vi "Log Response Times.vi"() -> ()   [LabVIEW 2015]
uses:
  <vilib>/addons/zeromq/socket_type.ctl
  <userlib>/_OpenG.lib/array/array.llb/Delete Elements from 1D Array (DBL)__ogtk.vi
  <vilib>/Utility/file.llb/Write Delimited Spreadsheet (string).vi
  <vilib>/addons/zeromq/zmq_context.lvclass
  <vilib>/addons/zeromq/zeromq.lvlib
  <vilib>/addons/zeromq/zmq_socket.lvclass
panel:
  out "Event Read Times":cluster{dbl[], i32[]}(graph)={[0.0009271277813240886, 0.2630802224110812, 0.5252333170408383, 0.7873864116705954, 1.0495395063003525, 1.3116926009301095, 1.5738456955598668, 1.835998790189624, 2.098151884819381, 2.360304979449138, 2.622458074078895, 2.8846111687086524, 3.1467642633384094, 3.4089173579681664, 3.671070452597924, 3.933223547227681, 4.195376641857438, 4.457529736487195, 4.719682831116952, 4.981835925746709, 5.243989020376466, 5.506142115006224, 5.768295209635981, 6.030448304265738, 6.292601398895495, 6.554754493525252, 6.816907588155009, 7.079060682784766, 7.341213777414524, 7.603366872044281, 7.865519966674038, 8.127673061303794, 8.389826155933552, 8.65197925056331, 8.914132345193066, 9.176285439822824, 9.43843853445258, 9.700591629082338, 9.962744723712094, 10.224897818341852, 10.487050912971608, 10.749204007601366, 11.011357102231123, 11.27351019686088, 11.535663291490637, 11.797816386120394, 12.059969480750151, 12.322122575379908, 12.584275670009665, 12.846428764639423, 13.10858185926918, 13.370734953898937, 13.632888048528693, 13.895041143158451, 14.157194237788207, 14.419347332417965, 14.681500427047723, 14.94365352167748, 15.205806616307237, 15.467959710936993, 15.730112805566751, 15.992265900196507, 16.254418994826263, 16.516572089456023, 16.77872518408578, 17.040878278715535, 17.303031373345295, 17.56518446797505, 17.827337562604807, 18.089490657234563, 18.351643751864323, 18.61379684649408, 18.875949941123835, 19.138103035753595, 19.40025613038335, 19.662409225013107, 19.924562319642863, 20.186715414272623, 20.44886850890238, 20.711021603532135, 20.97317469816189, 21.23532779279165, 21.497480887421407, 21.759633982051163, 22.021787076680923, 22.28394017131068, 22.546093265940435, 22.80824636057019, 23.07039945519995, 23.332552549829707, 23.594705644459463, 23.856858739089223, 24.11901183371898, 24.381164928348735, 24.64331802297849, 24.90547111760825, 25.167624212238007, 25.429777306867763, 25.691930401497522, 25.95408349612728], [281, 0, 0, 2, 0, 0, 0, 0, 0, 0, 1, 1, 1, 4, 11, 42, 21, 22, 12, 28, 8, 21, 11, 13, 18, 15, 90, 33, 52, 42, 68, 35, 22, 24, 110, 9, 3, 4, 4, 0, 1, 7, 1, 2, 0, 1, 0, 0, 0, 2, 0, 0, 0, 0, 0, 0, 0, 0, 0, 1, 0, 0, 0, 2, 0, 0, 1, 0, 2, 3, 0, 1, 3, 0, 1, 0, 0, 0, 0, 0, 0, 0, 0, 0, 0, 0, 0, 0, 1, 0, 0, 0, 0, 0, 0, 1, 0, 0, 0, 0]}
  out "Error Read Times":cluster{dbl[], i32[]}(graph)={[0.0009430865757167339, 0.30094855814939364, 0.6009540297230705, 0.9009595012967475, 1.2009649728704244, 1.5009704444441012, 1.8009759160177783, 2.100981387591455, 2.400986859165132, 2.700992330738809, 3.0009978023124857, 3.3010032738861628, 3.60100874545984, 3.9010142170335165, 4.201019688607193, 4.501025160180871, 4.801030631754547, 5.101036103328224, 5.401041574901901, 5.701047046475578, 6.001052518049255, 6.301057989622932, 6.601063461196609, 6.901068932770285, 7.201074404343963, 7.50107987591764, 7.801085347491316, 8.101090819064993, 8.40109629063867, 8.701101762212348, 9.001107233786025, 9.301112705359701, 9.601118176933378, 9.901123648507054, 10.201129120080731, 10.501134591654408, 10.801140063228086, 11.101145534801763, 11.40115100637544, 11.701156477949116, 12.001161949522793, 12.30116742109647, 12.601172892670148, 12.901178364243824, 13.2011838358175, 13.501189307391178, 13.801194778964854, 14.10120025053853, 14.40120572211221, 14.701211193685886, 15.001216665259562, 15.301222136833239, 15.601227608406916, 15.901233079980592, 16.20123855155427, 16.501244023127946, 16.801249494701622, 17.1012549662753, 17.40126043784898, 17.701265909422656, 18.001271380996332, 18.30127685257001, 18.601282324143686, 18.901287795717362, 19.20129326729104, 19.501298738864715, 19.801304210438392, 20.10130968201207, 20.401315153585745, 20.701320625159422, 21.0013260967331, 21.30133156830678, 21.601337039880455, 21.901342511454132, 22.20134798302781, 22.501353454601485, 22.801358926175162, 23.10136439774884, 23.401369869322515, 23.701375340896192, 24.00138081246987, 24.301386284043545, 24.60139175561722, 24.9013972271909, 25.20140269876458, 25.501408170338255, 25.80141364191193, 26.10141911348561, 26.401424585059285, 26.70143005663296, 27.00143552820664, 27.301440999780315, 27.60144647135399, 27.901451942927668, 28.201457414501345, 28.50146288607502, 28.8014683576487, 29.10147382922238, 29.401479300796055, 29.70148477236973], [281, 3, 0, 1, 0, 0, 0, 0, 0, 0, 3, 6, 4, 47, 33, 22, 47, 11, 11, 21, 8, 12, 25, 101, 51, 61, 65, 38, 35, 107, 13, 8, 3, 0, 1, 0, 4, 2, 0, 0, 0, 0, 0, 1, 0, 0, 1, 0, 0, 0, 0, 0, 1, 0, 0, 0, 1, 1, 1, 1, 0, 0, 0, 1, 0, 1, 0, 1, 0, 0, 0, 0, 0, 0, 0, 0, 0, 0, 0, 0, 0, 1, 0, 1, 0, 0, 0, 0, 0, 2, 0, 0, 0, 0, 0, 0, 0, 0, 0, 0]}
  in  "READ":bool
  in  "Error Log Request":string="{\"msg_id\":\"666\",\"msg_type\":\"get\",\"msg_property\":\"error\",\"XXX\":\"XXX\"}"
  in  "Event Log Request":string="{\"msg_id\":\"555\",\"msg_type\":\"get\",\"msg_property\":\"event\",\"XXX\":\"XXX\"}"
  in  "Message":string="{\"msg_id\":\"555\",\"msg_type\":\"read\",\"msg_property\":\"vmon\",\"8-04\":\"XXX\"}"
  in  "timeout (ms)":i32=1000
  in  "file":path=path "C:/Users/ANNIE/Documents/Logs/ZMQ_Read_Times.csv"
  in  "SEND":bool
  out "HB":bool
  out "error out":errorcluster
  in  "stop":bool
  in  "ZMQ endpoint":string="tcp://127.0.0.1:5555"
  out "REPLY":string
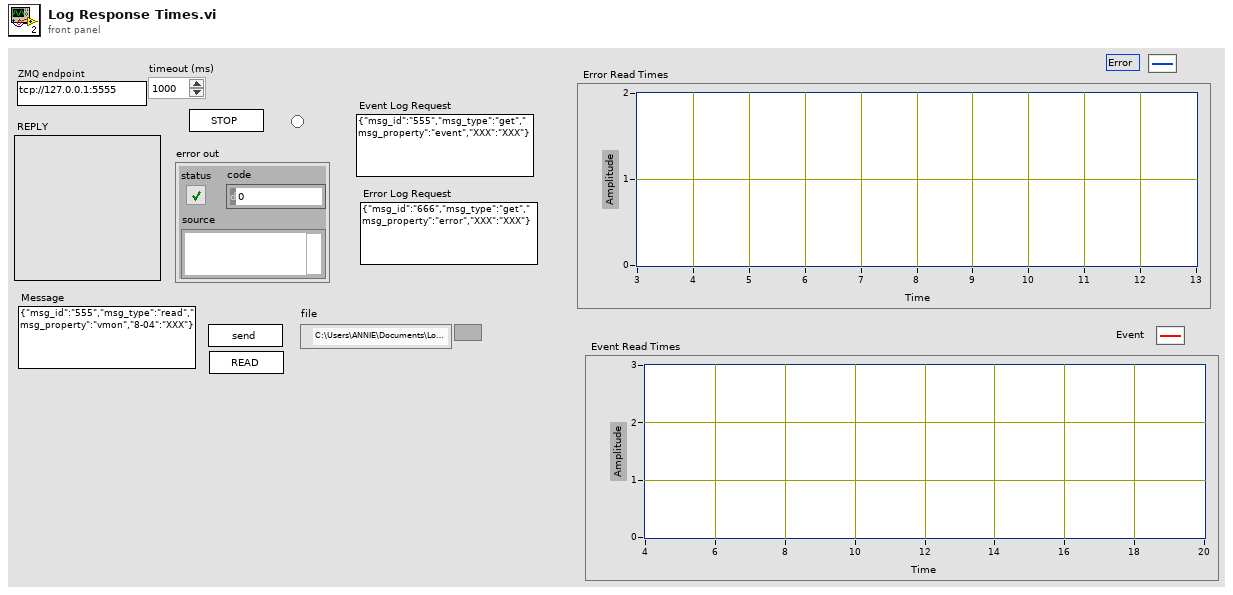
[diagram p1: front panel]
types:
  T1 = typedef "zeromq.lvlib/socket_type.ctl" = enum8{"ZMQ_PAIR", "ZMQ_PUB", "ZMQ_SUB", "ZMQ_REQ", "ZMQ_REP", "ZMQ_DEALER", "ZMQ_ROUTER", "ZMQ_PULL", "ZMQ_PUSH", "ZMQ_XPUB", "ZMQ_XSUB"}
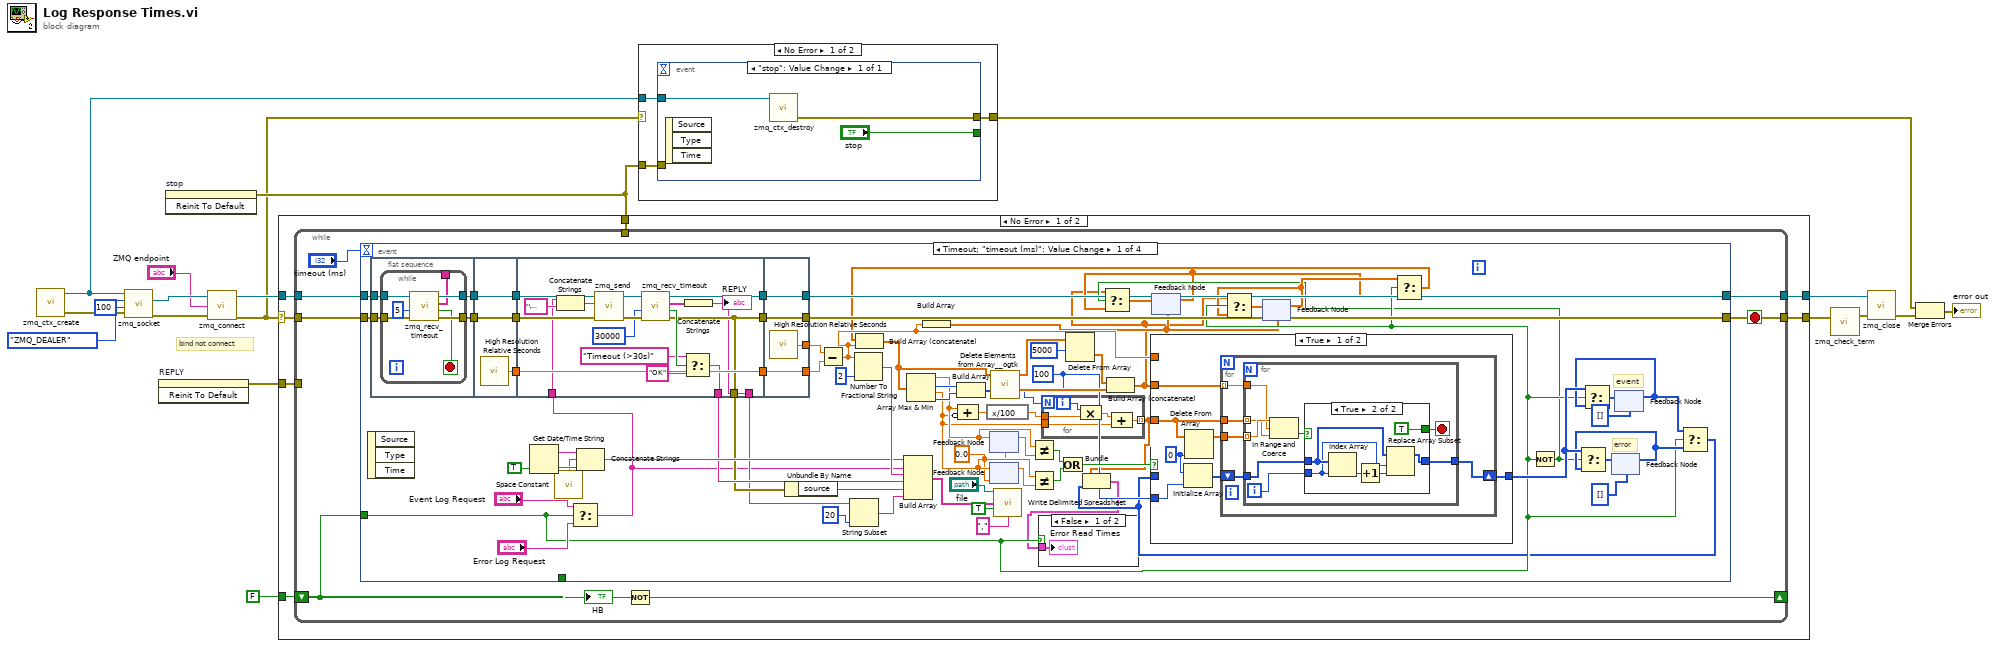
[diagram p0: block diagram]
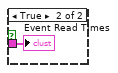
[diagram p2: hidden frame]
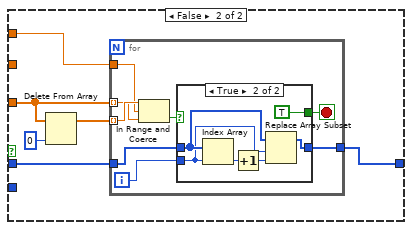
[diagram p4: hidden frame]
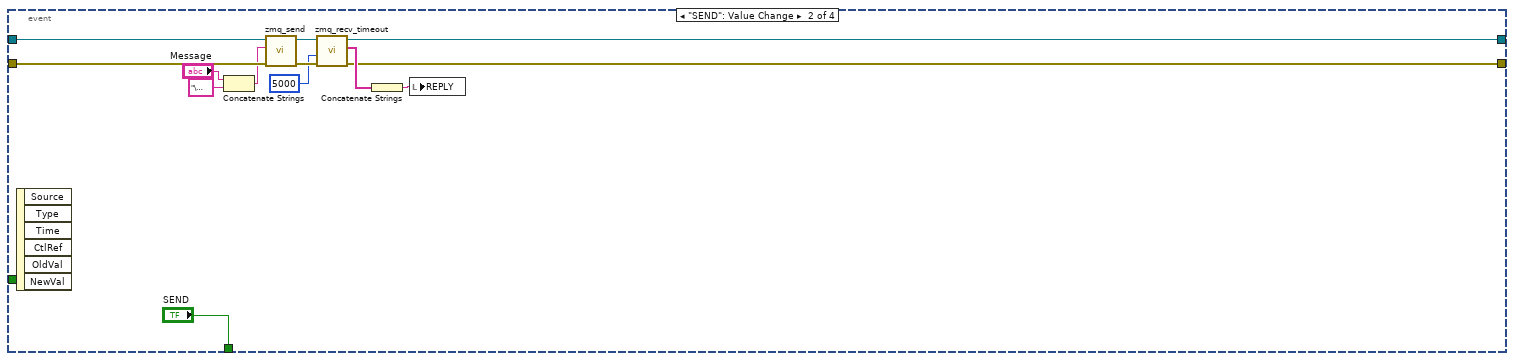
[diagram p6: hidden frame]
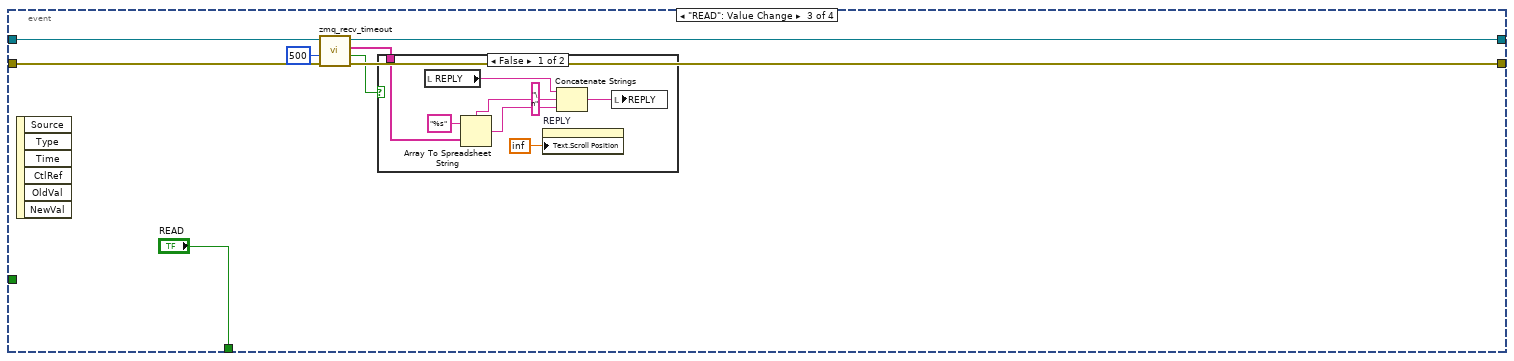
[diagram p7: hidden frame]
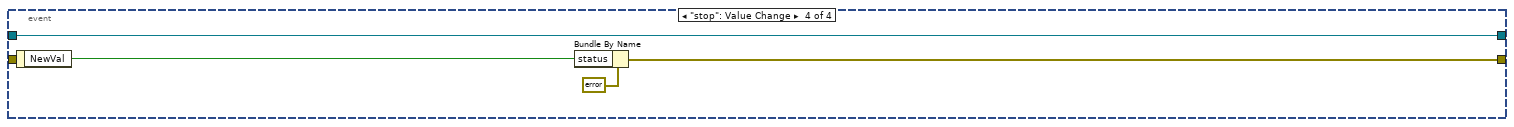
[diagram p9: hidden frame]
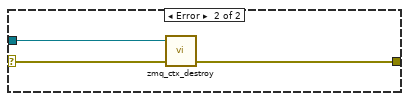
[diagram p11: hidden frame]
diagram:
  # "bind not connect"
  n1 = call <vilib>:"zmq_ctx_create.vi"() -> ("error out"=w12:errorcluster, "context out"=w10:refnum<class "zmq_context.lvclass">)  [unwired: 4 in]
  n2 = call <vilib>:"zmq_socket.vi"("error in"=w12, "linger (ms)"=100, "socket type"=socket_type."ZMQ_DEALER", "context in"=w10) -> ("error out"=w16:errorcluster, "socket out"=w17:refnum<class "zmq_socket.lvclass">)  [unwired: 1 in, 1 out]
  n3 = invoke on="REPLY" class="Str" method="Reinit To Default"() -> (error out=w11:errorcluster)  [unwired: 3 in, 2 out]
  n4 = invoke on="stop" class="Bool" method="Reinit To Default"() -> (error out=w3:errorcluster)  [unwired: 3 in, 2 out]
  n5 = call <vilib>:"zmq_connect.vi"("error in"=w16, "endpoint"="ZMQ endpoint", "socket in"=w17) -> ("error out"=w1:errorcluster, "socket out"=w15:refnum<class "zmq_socket.lvclass">)  [unwired: 1 in]
  n6 = case shown="No Error" w1 {
    selector: w1 -> [w19 w229]
    tunnel: w15 -> [w25 w228]
    tunnel: [w24 w228] -> w14
    tunnel: w11 -> [w23 _]
    tunnel: [w22 w229] -> w9
    tunnel: FALSE ("stop") -> [w21 _]
    tunnel: w3 -> [w20 _]
    frame No Error {
      n7 = while {
        tunnel: w25 -> [w32]
        tunnel: w19 -> [w31]
        tunnel: [w30] -> w24
        tunnel: [w28] -> w22
        tunnel: w23 -> [_]
        shift-right: [w29] -> _
        shift-left: w21 -> [w26]
        tunnel: w20 -> [_]
        stop <- w28 stop-if-true
        n8 = event shown="[0] Timeout;  \"timeout (ms)\": Value Change" {
          selector: _ -> [_ _ _ _]
          dyn-events: _ -> [_ _ _ _]
          timeout: "timeout (ms)" -> [_ _ _ _]
          tunnel: w32 -> [w105 w208 w216 w227]
          tunnel: w31 -> [w104 w207 w215 _]
          tunnel: [w101 w198 w212 w227] -> w30
          tunnel: [w100 w197 w213 w225] -> w28
          tunnel: w26 -> [w46 _ _ _]
          tunnel: [_ "SEND" "READ" _] -> _
          event Timeout; "timeout (ms)": Value Change {
            w48 = 0.0 ("index")
            w61 = 100 ("index")
            # "error"
            # "event"
            n9 = event-data() -> ()  [unwired: 1 in, 3 out]
            n10 = flat-sequence {
              tunnel: w104 -> [w161]
              tunnel: w105 -> [w164]
              tunnel: [w163] -> w34
              tunnel: [w162] -> w33
              tunnel: [w174] -> w103
              tunnel: [w173] -> w102
              tunnel: [w172] -> w94
              tunnel: w34 -> [w174]
              tunnel: w33 -> [w173]
              tunnel: w102 -> [w185]
              tunnel: w103 -> [w186]
              tunnel: [w189] -> w99
              tunnel: [w177] -> w98
              tunnel: [w182] -> w95
              tunnel: w94 -> [w182]
              tunnel: [w178] -> w87
              tunnel: [w177] -> w86
              tunnel: [w176] -> w84
              tunnel: w57 -> [w175]
              tunnel: [w194] -> w100
              tunnel: [w195] -> w101
              tunnel: w99 -> [w195]
              tunnel: w98 -> [w194]
              tunnel: [w193] -> w97
              tunnel: [w192] -> w96
              tunnel: w95 -> [w192]
              frame #0 {
                n11 = while {
                  tunnel: w164 -> [w171]
                  tunnel: [w170] -> w163
                  tunnel: [w169] -> w162
                  tunnel: w161 -> [w168]
                  tunnel: [w166] -> _
                  stop <- w167 stop-if-true
                  n12 = call <vilib>:"zmq_recv_timeout.vi"("error in"=w168, "timeout (ms)"=u32 5, "socket in"=w171) -> ("error out"=w169:errorcluster, "timeout?"=w167:bool, "parts"=w166:string[], "socket out"=w170:refnum<class "zmq_socket.lvclass">)  [unwired: 1 in]
                }
              }
              frame #1 {
                n13 = call <vilib>:"High Resolution Relative Seconds.vi"() -> ("relative seconds"=w172:dbl)
              }
              frame #2 {
                n14 = Concatenate Strings(w175, "\u0000" ("string")) -> (w183:string)
                n15 = call <vilib>:"zmq_send.vi"("error in"=w185, "data"=w183, "socket in"=w186) -> ("error out"=w188:errorcluster, "socket out"=w190:refnum<class "zmq_socket.lvclass">)  [unwired: 4 in]
                n16 = call <vilib>:"zmq_recv_timeout.vi"("error in"=w188, "timeout (ms)"=u32 30000, "socket in"=w190) -> ("error out"=w177:errorcluster, "timeout?"=w181:bool, "parts"=w191:string[], "socket out"=w189:refnum<class "zmq_socket.lvclass">)  [unwired: 1 in]
                n17 = Select(t="Timeout (>30s)" ("string"), s=w181, f="OK" ("string")) -> (s? t:f=w178:string)
                n18 = Concatenate Strings(w191) -> (w176:string)
                "REPLY" <- w176
              }
              frame #3 {
                n19 = call <vilib>:"High Resolution Relative Seconds.vi"() -> ("relative seconds"=w193:dbl)
              }
            }
            n20 = Get Date/Time String(want seconds? (F)=TRUE) -> (date string=w93:string, time string=w92:string)  [unwired: 2 in]
            n21 = call <vilib>:"Space Constant.vi"() -> ("String"=w91:string)
            n22 = Select(t="Event Log Request", s=w46, f="Error Log Request") -> (s? t:f=w57:string)
            n23 = Concatenate Strings(w93, w91, w92) -> (w88:string)
            n24 = Unbundle By Name(w86) -> ("source"=w85:string)
            n25 = Subtract(x=w97, y=w96) -> (x-y=w47:dbl)
            n26 = String Subset(string=w84, length (rest)=20 ("length (rest)")) -> (substring=w82:string)  [unwired: 1 in]
            n27 = Number To Fractional String(number=w47, precision (6)=i16 2) -> (F-format string=w89:string)  [unwired: 2 in]
            n28 = Build Array(w88, w57, w89, w87, w85, w82) -> (w81:string[])
            n29 = Build Array(w47) -> (w41:dbl[])
            n30 = feedback #1(w48) -> (w68:dbl)
            n31 = feedback #2(w48) -> (w65:dbl)
            n32 = call-poly <vilib>:"Write Delimited Spreadsheet.vi"("file path (dialog if empty)"="file", "1D data"=w81, "append to file? (F)"=TRUE, "delimiter (\\t)"="," ("delimiter (\\t)")) -> ()  [unwired: 10 in, 2 out]
            n33 = feedback #3(w41) -> (w39:dbl[])
            n34 = feedback #4(w41) -> (w44:dbl[])
            n35 = Select(t=w44, s=w46, f=w39) -> (s? t:f=w43:dbl[])
            n36 = Build Array (concatenate)(w43, w47) -> (w79:dbl[])
            n37 = Array Max & Min(array=w79) -> (max value=w67:dbl, max index (indices)=w77:i32, min value=w66:dbl, min index (indices)=w76:i32)
            n38 = Build Array(w77, w76) -> (w78:i32[])
            n39 = Compound Arithmetic op=ADD(w67, invert w66) -> (w69:dbl)
            n40 = expression code="x/100"(w69) -> (w72:dbl)
            n41 = feedback-in #1(w67) -> ()
            n42 = feedback-in #2(w66) -> ()
            n43 = call-poly <userlib>:"Delete Elements from Array__ogtk.vi"("indices"=w78, "array"=w79) -> ("deleted elements"=w73:dbl[], "array w/ subset deleted"=w75:dbl[])  [unwired: 8 in]
            n44 = Not Equal?(x=w67, y=w68) -> (x != y?=w64:bool)
            n45 = Not Equal?(x=w66, y=w65) -> (x != y?=w63:bool)
            n46 = for {
              N: w61 -> [_]
              tunnel: w72 -> [w160]
              tunnel: w66 -> [w157]
              tunnel: [w156] -> w35 mode=indexing
              i -> [w159]
              n47 = Compound Arithmetic op=MULTIPLY(w159, w160) -> (w158:dbl)
              n48 = Compound Arithmetic op=ADD(w158, w157) -> (w156:dbl)
            }
            n49 = Or(x=w64, y=w63) -> (x .or. y?=w62:bool)
            n50 = Delete From Array(array=w75, length=5000) -> (deleted portion=w74:dbl[])  [unwired: 1 in, 1 out]
            n51 = Build Array (concatenate)(w74, w73) -> (w38:dbl[])
            n52 = Select(t=w38, s=w46, f=w44) -> (s? t:f=w45:dbl[])
            n53 = feedback-in #4(w45) -> ()
            n54 = Not(x=w46) -> (.not. x?=w42:bool)
            n55 = Select(t=w38, s=w42, f=w39) -> (s? t:f=w40:dbl[])
            n56 = feedback-in #3(w40) -> ()
            n57 = feedback #5(i32[] []) -> (w51:i32[])
            n58 = feedback #6(i32[] []) -> (w52:i32[])
            n59 = Select(t=w52, s=w46, f=w51) -> (s? t:f=w37:i32[])
            n60 = Bundle(w35, w37) -> (w36:cluster{dbl[], i32[]})  [unwired: 1 in]
            n61 = case shown="False" w46 {
              tunnel: w36 -> [w106 w107]
              frame False {
                "Error Read Times" <- w106
              }
              frame True {
                "Event Read Times" <- w107
              }
            }
            n62 = case shown="True" w62 {
              tunnel: w38 -> [w114 _]
              tunnel: w35 -> [w113 w140]
              tunnel: [w109 w137] -> w54
              tunnel: w37 -> [_ w136]
              tunnel: w47 -> [_ w135]
              tunnel: w61 -> [w108 _]
              frame True {
                w110 = 0 ("index")
                n63 = Initialize Array(w110, w108) -> (w111:i32[])
                n64 = Delete From Array(array=w113, index=w110) -> (array with subset deleted=w112:dbl[])  [unwired: 1 in, 1 out]
                n65 = for {
                  tunnel: w113 -> [w118]
                  tunnel: w114 -> [w119] mode=indexing
                  tunnel: w112 -> [w117]
                  shift-right: [w115] -> w109
                  shift-left: w111 -> [w116]
                  n66 = for {
                    tunnel: w119 -> [w125]
                    tunnel: w118 -> [w126] mode=indexing
                    tunnel: w117 -> [w127] mode=indexing
                    tunnel: w116 -> [w123]
                    tunnel: [w121] -> w115
                    i -> [w122]
                    stop <- w120 stop-if-true
                    n67 = In Range and Coerce(upper limit=w127, x=w125, lower limit=w126) -> (In Range?=w124:bool)  [unwired: 1 out]
                    n68 = case shown="True" w124 {
                      tunnel: w123 -> [w128 w132]
                      tunnel: w122 -> [_ w131]
                      tunnel: [w128 w130] -> w121
                      tunnel: [_ TRUE ("append to file? (F)")] -> w120
                      frame False {
                      }
                      frame True {
                        n69 = Index Array(array=w132, index=w131) -> (element=w134:i32)
                        n70 = Increment(x=w134) -> (x+1=w133:i32)
                        n71 = Replace Array Subset(array=w132, new element=w133, index=w131) -> (w130:i32[])
                      }
                    }
                  }
                }
              }
              frame False {
                n72 = Delete From Array(array=w140, index=0) -> (array with subset deleted=w139:dbl[])  [unwired: 1 in, 1 out]
                n73 = for {
                  tunnel: w135 -> [w146]
                  tunnel: w140 -> [w147] mode=indexing
                  tunnel: w139 -> [w148] mode=indexing
                  tunnel: w136 -> [w144]
                  tunnel: [w142] -> w137
                  i -> [w143]
                  stop <- w141 stop-if-true
                  n74 = In Range and Coerce(upper limit=w148, x=w146, lower limit=w147) -> (In Range?=w145:bool)  [unwired: 1 out]
                  n75 = case shown="True" w145 {
                    tunnel: w144 -> [w149 w153]
                    tunnel: w143 -> [_ w152]
                    tunnel: [w149 w151] -> w142
                    tunnel: [_ TRUE ("append to file? (F)")] -> w141
                    frame False {
                    }
                    frame True {
                      n76 = Index Array(array=w153, index=w152) -> (element=w155:i32)
                      n77 = Increment(x=w155) -> (x+1=w154:i32)
                      n78 = Replace Array Subset(array=w153, new element=w154, index=w152) -> (w151:i32[])
                    }
                  }
                }
              }
            }
            n79 = Select(t=w54, s=w42, f=w51) -> (s? t:f=w53:i32[])
            n80 = Select(t=w54, s=w46, f=w52) -> (s? t:f=w55:i32[])
            n81 = feedback-in #5(w53) -> ()
            n82 = feedback-in #6(w55) -> ()
          }
          event "SEND": Value Change {
            n83 = event-data() -> ()  [unwired: 1 in, 6 out]
            n84 = Concatenate Strings("Message", "\u0000" ("string")) -> (w200:string)
            n85 = call <vilib>:"zmq_send.vi"("error in"=w207, "data"=w200, "socket in"=w208) -> ("error out"=w204:errorcluster, "socket out"=w205:refnum<class "zmq_socket.lvclass">)  [unwired: 4 in]
            n86 = call <vilib>:"zmq_recv_timeout.vi"("error in"=w204, "timeout (ms)"=u32 5000, "socket in"=w205) -> ("error out"=w197:errorcluster, "parts"=w206:string[], "socket out"=w198:refnum<class "zmq_socket.lvclass">)  [unwired: 1 in, 1 out]
            n87 = Concatenate Strings(w206) -> (w199:string)
            n88 = local write "REPLY"(w199) -> ()
          }
          event "READ": Value Change {
            n89 = event-data() -> ()  [unwired: 1 in, 6 out]
            n90 = call <vilib>:"zmq_recv_timeout.vi"("error in"=w215, "timeout (ms)"=u32 500, "socket in"=w216) -> ("error out"=w213:errorcluster, "timeout?"=w210:bool, "parts"=w211:string[], "socket out"=w212:refnum<class "zmq_socket.lvclass">)  [unwired: 1 in]
            n91 = case shown="False" w210 {
              tunnel: w211 -> [w219 _]
              frame False {
                w220 = "\n" ("string")
                n92 = local read "REPLY"() -> (w222:string)
                n93 = Array To Spreadsheet String(delimiter (Tab)=w220, array=w219, 3:"%s" ("format string")) -> (spreadsheet string=w218:string)
                n94 = property on="REPLY" class="Str"("Text.Scroll Position"=inf) -> ()  [unwired: 2 in, 2 out]
                n95 = Concatenate Strings(w222, w220, w218) -> (w223:string)
                n96 = local write "REPLY"(w223) -> ()
              }
              frame True {
              }
            }
          }
          event "stop": Value Change {
            n97 = event-data() -> ("NewVal"=w226:bool)  [unwired: 1 in]
            n98 = Bundle By Name(cluster=errorcluster {"status"=FALSE, "code"=0, "source"=""} ("error out"), "status"=w226) -> (w225:errorcluster)
          }
        }
        n99 = Not(x=w26) -> (.not. x?=w29:bool)
        "HB" <- w26
      }
    }
    frame Error {
    }
  }
  n100 = case shown="No Error" w1 {
    selector: w1 -> [_ w237]
    tunnel: w10 -> [w232 w238]
    tunnel: [w231 w236] -> w6
    tunnel: w3 -> [w230 _]
    frame No Error {
      n101 = event shown="[0] \"stop\": Value Change" {
        selector: _ -> [_]
        dyn-events: _ -> [_]
        timeout: _ -> [_]
        tunnel: w232 -> [w235]
        tunnel: ["stop"] -> _
        tunnel: [w233] -> w231
        tunnel: w230 -> [_]
        event "stop": Value Change {
          n102 = event-data() -> ()  [unwired: 1 in, 3 out]
          n103 = call <vilib>:"zmq_ctx_destroy.vi"("context in"=w235) -> ("error out"=w233:errorcluster)  [unwired: 4 in]
        }
      }
    }
    frame Error {
      n104 = call <vilib>:"zmq_ctx_destroy.vi"("error in"=w237, "context in"=w238) -> ("error out"=w236:errorcluster)  [unwired: 3 in]
    }
  }
  n105 = call <vilib>:"zmq_check_term.vi"("error in"=w9) -> ("error out"=w8:errorcluster)  [unwired: 1 in, 1 out]
  n106 = call <vilib>:"zmq_close.vi"("error in"=w8, "socket"=w14) -> ("error out"=w7:errorcluster)  [unwired: 3 in]
  n107 = Merge Errors(w6, w7) -> (→"error out":errorcluster)
